vi "Weather Parse Test.vi"() -> ()   [LabVIEW 2020, in "CDM-Config.lvlib"] (continued)
                  \"SUY\"\n                    ]\n                }\n            }\n        },\n        {\n            \"id\": \"https://api.weather.gov/alerts/urn:oid:2.49.0.1.840.0.13e054451602e8337e1efcccba613b86623b52ca.001.1\",\n            \"type\": \"Feature\",\n            \"geometry\": null,\n            \"properties\": {\n                \"@id\": \"https://api.weather.gov/alerts/urn:oid:2.49.0.1.840.0.13e054451602e8337e1efcccba613b86623b52ca.001.1\",\n                \"@type\": \"wx:Alert\",\n                \"id\": \"urn:oid:2.49.0.1.840.0.13e054451602e8337e1efcccba613b86623b52ca.001.1\",\n                \"areaDesc\": \"Cimarron; Texas; Dallam; Sherman; Hansford; Hartley; Moore; Hutchinson; Oldham; Potter; Carson; Deaf Smith; Randall; Armstrong; Palo Duro Canyon\",\n                \"geocode\": {\n                    \"SAME\": [\n                        \"040025\",\n                        \"040139\",\n                        \"048111\",\n                        \"048421\",\n                        \"048195\",\n                        \"048205\",\n                        \"048341\",\n                        \"048233\",\n                        \"048359\",\n                        \"048375\",\n                        \"048065\",\n                        \"048117\",\n                        \"048381\",\n                        \"048011\"\n                    ],\n                    \"UGC\": [\n                        \"OKZ001\",\n                        \"OKZ002\",\n                        \"TXZ001\",\n                        \"TXZ002\",\n                        \"TXZ003\",\n                        \"TXZ006\",\n                        \"TXZ007\",\n                        \"TXZ008\",\n                        \"TXZ011\",\n                        \"TXZ012\",\n                        \"TXZ013\",\n                        \"TXZ016\",\n                        \"TXZ017\",\n                        \"TXZ018\",\n                        \"TXZ317\"\n                    ]\n                },\n                \"affectedZones\": [\n                    \"https://api.weather.gov/zones/forecast/OKZ001\",\n                    \"https://api.weather.gov/zones/forecast/OKZ002\",\n                    \"https://api.weather.gov/zones/forecast/TXZ001\",\n                    \"https://api.weather.gov/zones/forecast/TXZ002\",\n                    \"https://api.weather.gov/zones/forecast/TXZ003\",\n                    \"https://api.weather.gov/zones/forecast/TXZ006\",\n                    \"https://api.weather.gov/zones/forecast/TXZ007\",\n                    \"https://api.weather.gov/zones/forecast/TXZ008\",\n                    \"https://api.weather.gov/zones/forecast/TXZ011\",\n                    \"https://api.weather.gov/zones/forecast/TXZ012\",\n                    \"https://api.weather.gov/zones/forecast/TXZ013\",\n                    \"https://api.weather.gov/zones/forecast/TXZ016\",\n                    \"https://api.weather.gov/zones/forecast/TXZ017\",\n                    \"https://api.weather.gov/zones/forecast/TXZ018\",\n                    \"https://api.weather.gov/zones/forecast/TXZ317\"\n                ],\n                \"references\": [],\n                \"sent\": \"2025-12-02T22:29:00-06:00\",\n                \"effective\": \"2025-12-02T22:29:00-06:00\",\n                \"onset\": \"2025-12-02T22:29:00-06:00\",\n                \"expires\": \"2025-12-03T12:00:00-06:00\",\n                \"ends\": null,\n                \"status\": \"Actual\",\n                \"messageType\": \"Alert\",\n                \"category\": \"Met\",\n                \"severity\": \"Moderate\",\n                \"certainty\": \"Observed\",\n                \"urgency\": \"Expected\",\n                \"event\": \"Special Weather Statement\",\n                \"sender\": \"w-nws.webmaster@noaa.gov\",\n                \"senderName\": \"NWS Amarillo TX\",\n                \"headline\": \"Special Weather Statement issued December 2 at 10:29PM CST by NWS Amarillo TX\",\n                \"description\": \"Winter weather is on the way to the Panhandles Wednesday afternoon\\ninto Thursday. A weather system is expected to move over the Four\\nCorners Wednesday and then track east across New Mexico on\\nWednesday night. Out ahead of this system a strong cold front,\\nassociated with a much larger cold air mass over Canada will bring\\ncold enough temperatures to the Panhandles to allow the\\nprecipitation to be in the form of snow.\\n\\nIt's anticipated that this system will produce some snow bands,\\npossibly a narrow area of snow. These band locations could range\\nfrom the Oklahoma Panhandle down to the southern Texas Panhandle.\\nRight now there's high uncertainty on the location of the snow\\nbands, so much that winter highlights are currently on hold. As\\nthe system approaches and we narrow down the areas that have the\\ngreatest chances of impactful accumulating snow, then we'll add\\nwinter highlights as needed.\\n\\nRight now areas covered in this statement have about a 30 to 60\\npercent chance of receiving at least an inch of snow between\\nWednesday afternoon, and Thursday evening. But if these turn out\\nto be narrow snow bands, then there could be several areas that\\nreceive little to no snow, while more isolated areas pick up 1 to\\n2 inches of snow. And those same areas would have about a 10\\npercent chance of greater than 2 inches of snow.\\n\\nAs it stands right now the best chance for snow to occur in\\nOklahoma to northwest Texas would be mid day Wednesday through\\nmidnight Wednesday night. West of Amarillo to Guymon has the best\\nchance for snow from 9PM Wednesday through about 6 AM Thursday\\nmorning. And east of that same line would be from 3AM to 3PM\\nThursday.\",\n                \"instruction\": null,\n                \"response\": \"Execute\",\n                \"parameters\": {\n                    \"AWIPSidentifier\": [\n                        \"SPSAMA\"\n                    ],\n                    \"WMOidentifier\": [\n                        \"WWUS84 KAMA 030429\"\n                    ],\n                    \"BLOCKCHANNEL\": [\n                        \"EAS\",\n                        \"NWEM\",\n                        \"CMAS\"\n                    ],\n                    \"EAS-ORG\": [\n                        \"WXR\"\n                    ]\n                },\n                \"scope\": \"Public\",\n                \"code\": \"IPAWSv1.0\",\n                \"language\": \"en-US\",\n                \"web\": \"http://www.weather.gov\",\n                \"eventCode\": {\n                    \"SAME\": [\n                        \"SPS\"\n                    ],\n                    \"NationalWeatherService\": [\n                        \"SPS\"\n                    ]\n                }\n            }\n        },\n        {\n            \"id\": \"https://api.weather.gov/alerts/urn:oid:2.49.0.1.840.0.4a77df2fdf2b5a368cb145dcee20e0db7f971925.002.1\",\n            \"type\": \"Feature\",\n            \"geometry\": null,\n            \"properties\": {\n                \"@id\": \"https://api.weather.gov/alerts/urn:oid:2.49.0.1.840.0.4a77df2fdf2b5a368cb145dcee20e0db7f971925.002.1\",\n                \"@type\": \"wx:Alert\",\n                \"id\": \"urn:oid:2.49.0.1.840.0.4a77df2fdf2b5a368cb145dcee20e0db7f971925.002.1\",\n                \"areaDesc\": \"Majuro\",\n                \"geocode\": {\n                    \"SAME\": [\n                        \"068190\"\n                    ],\n                    \"UGC\": [\n                        \"MHZ002\"\n                    ]\n                },\n                \"affectedZones\": [\n                    \"https://api.weather.gov/zones/forecast/MHZ002\"\n                ],\n                \"references\": [\n                    {\n                        \"@id\": \"https://api.weather.gov/alerts/urn:oid:2.49.0.1.840.0.fd750872e36744c34b2c9a183ece0ba44d257df6.002.1\",\n                        \"identifier\": \"urn:oid:2.49.0.1.840.0.fd750872e36744c34b2c9a183ece0ba44d257df6.002.1\",\n                        \"sender\": \"w-nws.webmaster@noaa.gov\",\n                        \"sent\": \"2025-12-03T02:41:00+10:00\"\n                    }\n                ],\n                \"sent\": \"2025-12-03T14:00:00+10:00\",\n                \"effective\": \"2025-12-03T14:00:00+10:00\",\n                \"onset\": \"2025-12-03T14:00:00+10:00\",\n                \"expires\": \"2025-12-04T04:00:00+10:00\",\n                \"ends\": \"2025-12-05T16:00:00+10:00\",\n                \"status\": \"Actual\",\n                \"messageType\": \"Update\",\n                \"category\": \"Met\",\n                \"severity\": \"Minor\",\n                \"certainty\": \"Likely\",\n                \"urgency\": \"Expected\",\n                \"event\": \"Coastal Flood Statement\",\n                \"sender\": \"w-nws.webmaster@noaa.gov\",\n                \"senderName\": \"NWS Tiyan GU\",\n                \"headline\": \"Coastal Flood Statement issued December 3 at 2:00PM ChST until December 5 at 4:00PM ChST by NWS Tiyan GU\",\n                \"description\": \"* WHAT...Isolated minor coastal flooding.\\n\\n* WHERE...North and east facing shorelines of Majuro.\\n\\n* WHEN...Through Friday afternoon.\\n\\n* IMPACTS...Some water on low lying roads and property.\\n\\n* ADDITIONAL DETAILS...Tide predictions show increasing wave run\\nup across Majuro this week due a combination of the lunar cycle\\nand a north swell from a distant weather system. Isolated minor\\ncoastal flooding is expected through at least Friday afternoon.\",\n                \"instruction\": \"Watch for debris along low-lying shorelines facing north and\\neast. Residents living along these low-lying shorelines need to\\nmonitor water levels and take actions to protect property from\\ninundation.\",\n                \"response\": \"Monitor\",\n                \"parameters\": {\n                    \"AWIPSidentifier\": [\n                        \"CFWPQ1\"\n                    ],\n                    \"WMOidentifier\": [\n                        \"WHPQ41 PGUM 030400\"\n                    ],\n                    \"NWSheadline\": [\n                        \"COASTAL FLOOD STATEMENT REMAINS IN EFFECT THROUGH FRIDAY AFTERNOON\"\n                    ],\n                    \"BLOCKCHANNEL\": [\n                        \"EAS\",\n                        \"NWEM\",\n                        \"CMAS\"\n                    ],\n                    \"VTEC\": [\n                        \"/O.CON.PGUM.CF.S.0005.000000T0000Z-251205T0600Z/\"\n                    ],\n                    \"eventEndingTime\": [\n                        \"2025-12-05T16:00:00+10:00\"\n                    ],\n                    \"expiredReferences\": [\n                        \"w-nws.webmaster@noaa.gov,urn:oid:2.49.0.1.840.0.2957d64b6528fdd549b26b0c52e7b17bd496878e.002.1,2025-12-02T14:18:00+10:00 w-nws.webmaster@noaa.gov,urn:oid:2.49.0.1.840.0.d051583a0fc14d57e91ab759b3686451f43fae66.002.1,2025-12-02T03:10:00+10:00 w-nws.webmaster@noaa.gov,urn:oid:2.49.0.1.840.0.3733fd1269a79576a68bee5bf75b40d4db85707a.002.1,2025-12-01T15:08:00+10:00\"\n                    ]\n                },\n                \"scope\": \"Public\",\n                \"code\": \"IPAWSv1.0\",\n                \"language\": \"en-US\",\n                \"web\": \"http://www.weather.gov\",\n                \"eventCode\": {\n                    \"SAME\": [\n                        \"NWS\"\n                    ],\n                    \"NationalWeatherService\": [\n                        \"CFS\"\n                    ]\n                }\n            }\n        },\n        {\n            \"id\": \"https://api.weather.gov/alerts/urn:oid:2.49.0.1.840.0.4a77df2fdf2b5a368cb145dcee20e0db7f971925.001.1\",\n            \"type\": \"Feature\",\n            \"geometry\": null,\n            \"properties\": {\n                \"@id\": \"https://api.weather.gov/alerts/urn:oid:2.49.0.1.840.0.4a77df2fdf2b5a368cb145dcee20e0db7f971925.001.1\",\n                \"@type\": \"wx:Alert\",\n                \"id\": \"urn:oid:2.49.0.1.840.0.4a77df2fdf2b5a368cb145dcee20e0db7f971925.001.1\",\n                \"areaDesc\": \"Kosrae; Pohnpei\",\n                \"geocode\": {\n                    \"SAME\": [\n                        \"064005\",\n                        \"064040\"\n                    ],\n                    \"UGC\": [\n                        \"FMZ001\",\n                        \"FMZ013\"\n                    ]\n                },\n                \"affectedZones\": [\n                    \"https://api.weather.gov/zones/forecast/FMZ001\",\n                    \"https://api.weather.gov/zones/forecast/FMZ013\"\n                ],\n                \"references\": [\n                    {\n                        \"@id\": \"https://api.weather.gov/alerts/urn:oid:2.49.0.1.840.0.fd750872e36744c34b2c9a183ece0ba44d257df6.001.1\",\n                        \"identifier\": \"urn:oid:2.49.0.1.840.0.fd750872e36744c34b2c9a183ece0ba44d257df6.001.1\",\n                        \"sender\": \"w-nws.webmaster@noaa.gov\",\n                        \"sent\": \"2025-12-03T02:41:00+10:00\"\n                    }\n                ],\n                \"sent\": \"2025-12-03T14:00:00+10:00\",\n                \"effective\": \"2025-12-03T14:00:00+10:00\",\n                \"onset\": \"2025-12-03T14:00:00+10:00\",\n                \"expires\": \"2025-12-04T04:00:00+10:00\",\n                \"ends\": \"2025-12-05T16:00:00+10:00\",\n                \"status\": \"Actual\",\n                \"messageType\": \"Update\",\n                \"category\": \"Met\",\n                \"severity\": \"Minor\",\n                \"certainty\": \"Likely\",\n                \"urgency\": \"Expected\",\n                \"event\": \"High Surf Advisory\",\n                \"sender\": \"w-nws.webmaster@noaa.gov\",\n                \"senderName\": \"NWS Tiyan GU\",\n                \"headline\": \"High Surf Advisory issued December 3 at 2:00PM ChST until December 5 at 4:00PM ChST by NWS Tiyan GU\",\n                \"description\": \"* WHAT...Large breaking waves of 7 to 10 feet.\\n\\n* WHERE...North and east facing reefs of Kosrae. North facing\\nreefs of Pohnpei.\\n\\n* WHEN...Until 4 PM ChST Friday.\\n\\n* IMPACTS...Dangerous swimming and surfing conditions and\\nlocalized beach erosion.\\n\\n* ADDITIONAL DETAILS...A long period northerly swell emanating\\nfrom a distant weather system combined with a large northeast\\ntrade swell continue to produce hazardous surf conditions for\\nPohnpei and Kosrae. Surf conditions look to remain hazardous\\nthrough at least Friday afternoon.\",\n                \"instruction\": \"Inexperienced swimmers should remain out of the water due to\\ndangerous surf conditions.\",\n                \"response\": \"Avoid\",\n                \"parameters\": {\n                    \"AWIPSidentifier\": [\n                        \"CFWPQ1\"\n                    ],\n                    \"WMOidentifier\": [\n                        \"WHPQ41 PGUM 030400\"\n                    ],\n                    \"NWSheadline\": [\n                        \"HIGH SURF ADVISORY NOW IN EFFECT UNTIL 4 PM CHST FRIDAY\"\n                    ],\n                    \"BLOCKCHANNEL\": [\n                        \"EAS\",\n                        \"NWEM\",\n                        \"CMAS\"\n                    ],\n                    \"VTEC\": [\n                        \"/O.EXT.PGUM.SU.Y.0038.000000T0000Z-251205T0600Z/\"\n                    ],\n                    \"eventEndingTime\": [\n                        \"2025-12-05T16:00:00+10:00\"\n                    ],\n                    \"expiredReferences\": [\n                        \"w-nws.webmaster@noaa.gov,urn:oid:2.49.0.1.840.0.2957d64b6528fdd549b26b0c52e7b17bd496878e.001.1,2025-12-02T14:18:00+10:00 w-nws.webmaster@noaa.gov,urn:oid:2.49.0.1.840.0.d051583a0fc14d57e91ab759b3686451f43fae66.001.1,2025-12-02T03:10:00+10:00 w-nws.webmaster@noaa.gov,urn:oid:2.49.0.1.840.0.3733fd1269a79576a68bee5bf75b40d4db85707a.001.1,2025-12-01T15:08:00+10:00\"\n                    ]\n                },\n                \"scope\": \"Public\",\n                \"code\": \"IPAWSv1.0\",\n                \"language\": \"en-US\",\n                \"web\": \"http://www.weather.gov\",\n                \"eventCode\": {\n                    \"SAME\": [\n                        \"NWS\"\n                    ],\n                    \"NationalWeatherService\": [\n                        \"SUY\"\n                    ]\n                }\n            }\n        },\n        {\n            \"id\": \"https://api.weather.gov/alerts/urn:oid:2.49.0.1.840.0.93baf164a8b81bd591d12264ddf37071887c834c.001.1\",\n            \"type\": \"Feature\",\n            \"geometry\": null,\n            \"properties\": {\n                \"@id\": \"https://api.weather.gov/alerts/urn:oid:2.49.0.1.840.0.93baf164a8b81bd591d12264ddf37071887c834c.001.1\",\n                \"@type\": \"wx:Alert\",\n                \"id\": \"urn:oid:2.49.0.1.840.0.93baf164a8b81bd591d12264ddf37071887c834c.001.1\",\n                \"areaDesc\": \"Kuskokwim Valley West; Kuskokwim Valley East; Kuskokwim Delta Coast and Nunivak Island; Interior Kuskokwim Delta\",\n                \"geocode\": {\n                    \"SAME\": [\n                        \"002050\"\n                    ],\n                    \"UGC\": [\n                        \"AKZ752\",\n                        \"AKZ753\",\n                        \"AKZ755\",\n                        \"AKZ756\"\n                    ]\n                },\n                \"affectedZones\": [\n                    \"https://api.weather.gov/zones/forecast/AKZ752\",\n                    \"https://api.weather.gov/zones/forecast/AKZ753\",\n                    \"https://api.weather.gov/zones/forecast/AKZ755\",\n                    \"https://api.weather.gov/zones/forecast/AKZ756\"\n                ],\n                \"references\": [],\n                \"sent\": \"2025-12-02T18:07:00-09:00\",\n                \"effective\": \"2025-12-02T18:07:00-09:00\",\n                \"onset\": \"2025-12-02T18:07:00-09:00\",\n                \"expires\": \"2025-12-03T09:00:00-09:00\",\n                \"ends\": \"2025-12-03T09:00:00-09:00\",\n                \"status\": \"Actual\",\n                \"messageType\": \"Alert\",\n                \"category\": \"Met\",\n                \"severity\": \"Extreme\",\n                \"certainty\": \"Likely\",\n                \"urgency\": \"Expected\",\n                \"event\": \"Ice Storm Warning\",\n                \"sender\": \"w-nws.webmaster@noaa.gov\",\n                \"senderName\": \"NWS Anchorage AK\",\n                \"headline\": \"Ice Storm Warning issued December 2 at 6:07PM AKST until December 3 at 9:00AM AKST by NWS Anchorage AK\",\n                \"description\": \"* WHAT...Significant icing expected. Ice accumulations around three\\nquarters of an inch.\\n\\nBlizzard conditions with wind gusts 45 to 55 mph reducing\\nvisibilities to 1/4 mile or less for coastal communities. Total snow\\naccumulations 6 to 12 inches.\\n\\n* WHERE...Kuskokwim Delta, Kuskokwim Valley, including Bethel,\\nAniak, and Crooked Creek for the Ice Storm.\\n\\nCoastal Kuskokwim Delta, including Nunivak and Nelson Islands for\\nBlizzard conditions.\\n\\n* WHEN...Until 9 AM AKST Wednesday.\\n\\n* IMPACTS...Travel could be very difficult. Surfaces will likely\\nbecome slick and hazardous. Significant ice accumulation may cause\\npower outages.\\n\\n* ADDITIONAL DETAILS...Precipitation will remain all snow north and\\nwest of Bethel. North and west of this line is where the Blizzard\\nconditions are ongoing. South and east of this line is where the\\nfreezing rain and Ice Storm conditions are observed.\",\n                \"instruction\": \"An Ice Storm Warning means significant amounts of ice accumulation\\nwill make travel extremely hazardous. Travel is strongly\\ndiscouraged. If you must travel, keep an extra flashlight, food and\\nwater in your vehicle in case of an emergency. Snapped power lines\\nare also possible.\\n\\nPrepare for possible power outages.\",\n                \"response\": \"Avoid\",\n                \"parameters\": {\n                    \"AWIPSidentifier\": [\n                        \"WSWALU\"\n                    ],\n                    \"WMOidentifier\": [\n                        \"WWAK42 PAFC 030307\"\n                    ],\n                    \"NWSheadline\": [\n                        \"ICE STORM WARNING REMAINS IN EFFECT UNTIL 9 AM AKST WEDNESDAY\"\n                    ],\n                    \"BLOCKCHANNEL\": [\n                        \"EAS\",\n                        \"NWEM\",\n                        \"CMAS\"\n                    ],\n                    \"EAS-ORG\": [\n                        \"WXR\"\n                    ],\n                    \"VTEC\": [\n                        \"/O.CON.PAFC.IS.W.0001.000000T0000Z-251203T1800Z/\"\n                    ],\n                    \"eventEndingTime\": [\n                        \"2025-12-03T09:00:00-09:00\"\n                    ],\n                    \"expiredReferences\": [\n                        \"w-nws.webmaster@noaa.gov,urn:oid:2.49.0.1.840.0.157c6f2e53da98a274a7f19e61fa4d73bdd57178.001.1,2025-12-02T00:42:00-09:00 w-nws.webmaster@noaa.gov,urn:oid:2.49.0.1.840.0.9ea12a385b049ff9ed2921f4adaaa88d8666a4fc.001.1,2025-12-01T15:28:00-09:00 w-nws.webmaster@noaa.gov,urn:oid:2.49.0.1.840.0.06a0cb035223f236a02d184a1ba736560d41ecbc.001.1,2025-12-01T04:08:00-09:00 w-nws.webmaster@noaa.gov,urn:oid:2.49.0.1.840.0.f69cd697e861d099e81d8f76b79e96457dfc9a38.001.1,2025-11-30T21:45:00-09:00 w-nws.webmaster@noaa.gov,urn:oid:2.49.0.1.840.0.ccdfa33bcad75d3bc47e8857a243a2cb5db88702.001.2,2025-11-30T09:50:00-09:00\"\n                    ]\n                },\n                \"scope\": \"Public\",\n                \"code\": \"IPAWSv1.0\",\n                \"language\": \"en-US\",\n                \"web\": \"http://www.weather.gov\",\n                \"eventCode\": {\n                    \"SAME\": [\n                        \"WSW\"\n                    ],\n                    \"NationalWeatherService\": [\n                        \"ISW\"\n                    ]\n                }\n            }\n        },\n        {\n            \"id\": \"https://api.weather.gov/alerts/urn:oid:2.49.0.1.840.0.72e634b4e6e77a16c94a0f4f045ba7b0b7412415.001.1\",\n            \"type\": \"Feature\",\n            \"geometry\": null,\n            \"properties\": {\n                \"@id\": \"https://api.weather.gov/alerts/urn:oid:2.49.0.1.840.0.72e634b4e6e77a16c94a0f4f045ba7b0b7412415.001.1\",\n                \"@type\": \"wx:Alert\",\n                \"id\": \"urn:oid:2.49.0.1.840.0.72e634b4e6e77a16c94a0f4f045ba7b0b7412415.001.1\",\n                \"areaDesc\": \"Yukon Delta Coast; Lower Yukon River; Lower Yukon and Innoko Valleys; North Slopes of the Western Alaska Range; Upper Kuskokwim Valley\",\n                \"geocode\": {\n                    \"SAME\": [\n                        \"002158\",\n                        \"002290\"\n                    ],\n                    \"UGC\": [\n                        \"AKZ825\",\n                        \"AKZ826\",\n                        \"AKZ830\",\n                        \"AKZ851\",\n                        \"AKZ852\"\n                    ]\n                },\n                \"affectedZones\": [\n                    \"https://api.weather.gov/zones/forecast/AKZ825\",\n                    \"https://api.weather.gov/zones/forecast/AKZ826\",\n                    \"https://api.weather.gov/zones/forecast/AKZ830\",\n                    \"https://api.weather.gov/zones/forecast/AKZ851\",\n                    \"https://api.weather.gov/zones/forecast/AKZ852\"\n                ],\n                \"references\": [\n                    {\n                        \"@id\": \"https://api.weather.gov/alerts/urn:oid:2.49.0.1.840.0.34d9addf2f9305801f81e1a30a2fd898a36c56d1.001.1\",\n                        \"identifier\": \"urn:oid:2.49.0.1.840.0.34d9addf2f9305801f81e1a30a2fd898a36c56d1.001.1\",\n                        \"sender\": \"w-nws.webmaster@noaa.gov\",\n                        \"sent\": \"2025-12-02T14:06:00-09:00\"\n                    },\n                    {\n                        \"@id\": \"https://api.weather.gov/alerts/urn:oid:2.49.0.1.840.0.0c7829ccd4c9dcb93f8b1cc70bbc58a8100d270e.002.1\",\n                        \"identifier\": \"urn:oid:2.49.0.1.840.0.0c7829ccd4c9dcb93f8b1cc70bbc58a8100d270e.002.1\",\n                        \"sender\": \"w-nws.webmaster@noaa.gov\",\n                        \"sent\": \"2025-12-02T17:58:00-09:00\"\n                    }\n                ],\n                \"sent\": \"2025-12-02T17:59:00-09:00\",\n                \"effective\": \"2025-12-02T17:59:00-09:00\",\n                \"onset\": \"2025-12-02T17:59:00-09:00\",\n                \"expires\": \"2025-12-03T15:00:00-09:00\",\n                \"ends\": \"2025-12-03T15:00:00-09:00\",\n                \"status\": \"Actual\",\n                \"messageType\": \"Update\",\n                \"category\": \"Met\",\n                \"severity\": \"Severe\",\n                \"certainty\": \"Likely\",\n                \"urgency\": \"Expected\",\n                \"event\": \"Winter Storm Warning\",\n                \"sender\": \"w-nws.webmaster@noaa.gov\",\n                \"senderName\": \"NWS Fairbanks AK\",\n                \"headline\": \"Winter Storm Warning issued December 2 at 5:59PM AKST until December 3 at 3:00PM AKST by NWS Fairbanks AK\",\n                \"description\": \"* WHAT...Heavy mixed precipitation. Additional snow accumulations up\\nto 4 inches and ice accumulations around a light glaze. Winds\\ngusting as high as 40 mph.\\n\\n* WHERE...Lower Yukon River, Lower Yukon and Innoko Valleys, North\\nSlopes of the Western Alaska Range, Upper Kuskokwim Valley, and\\nYukon Delta Coast.\\n\\n* WHEN...Until 3 PM AKST Wednesday.\\n\\n* IMPACTS...Surfaces will likely become slick and hazardous.\\nSignificant ice accumulation may cause power outages. Plan on very\\ndifficult traveling conditions.\\n\\nAdditional Details...\\nPrecipitation will be mainly snow, with a chance of freezing rain\\nlingering from McGrath south to the Alaska Range. Blizzard\\nconditions are expected at times for Hooper Bay and Chevak.\\nPrecipitation will taper off on Wednesday morning. Skies clear and\\ntemperatures cool rapidly Wednesday night.\",\n                \"instruction\": \"If you must travel, keep an extra flashlight, food, and water in\\nyour vehicle in case of an emergency. The latest road conditions for\\nthe state you are calling from can be obtained by calling 5 1 1.\",\n                \"response\": \"Prepare\",\n                \"parameters\": {\n                    \"AWIPSidentifier\": [\n                        \"WSWWCZ\"\n                    ],\n                    \"WMOidentifier\": [\n                        \"WWAK42 PAFG 030259\"\n                    ],\n                    \"NWSheadline\": [\n                        \"WINTER STORM WARNING REMAINS IN EFFECT UNTIL 3 PM AKST WEDNESDAY\"\n                    ],\n                    \"BLOCKCHANNEL\": [\n                        \"EAS\",\n                        \"NWEM\",\n                        \"CMAS\"\n                    ],\n                    \"EAS-ORG\": [\n                        \"WXR\"\n                    ],\n                    \"VTEC\": [\n                        \"/O.CON.PAFG.WS.W.0016.000000T0000Z-251204T0000Z/\"\n                    ],\n                    \"eventEndingTime\": [\n                        \"2025-12-03T15:00:00-09:00\"\n                    ],\n                    \"expiredReferences\": [\n                        \"w-nws.webmaster@noaa.gov,urn:oid:2.49.0.1.840.0.3180dc61ca5a09497ed0209ae9ba5ca85fe9aa38.001.1,2025-12-01T14:18:00-09:00 w-nws.webmaster@noaa.gov,urn:oid:2.49.0.1.840.0.ce7a20a2b61779be608b2c765e4513dcaffa8902.001.1,2025-11-30T21:20:00-09:00 w-nws.webmaster@noaa.gov,urn:oid:2.49.0.1.840.0.9c226504b9ca64cc9a49e8dc3ca9fdc84fc4ba17.001.1,2025-11-30T18:03:00-09:00 w-nws.webmaster@noaa.gov,urn:oid:2.49.0.1.840.0.8f81aa3d43b03a8113b1ac64dd14a9f9aab497bb.001.1,2025-11-30T13:06:00-09:00 w-nws.webmaster@noaa.gov,urn:oid:2.49.0.1.840.0.bf2353bea365d572d4db55ee3da60224ffafc19c.001.1,2025-11-29T15:10:00-09:00 w-nws.webmaster@noaa.gov,urn:oid:2.49.0.1.840.0.7ae26db47c90a11c53b2cafe361544d352e847b0.001.2,2025-11-29T13:57:00-09:00\"\n                    ]\n                },\n                \"scope\": \"Public\",\n                \"code\": \"IPAWSv1.0\",\n                \"language\": \"en-US\",\n                \"web\": \"http://www.weather.gov\",\n                \"eventCode\": {\n                    \"SAME\": [\n                        \"WSW\"\n                    ],\n                    \"NationalWeatherService\": [\n                        \"WSW\"\n                    ]\n                }\n            }\n        },\n        {\n            \"id\": \"https://api.weather.gov/alerts/urn:oid:2.49.0.1.840.0.b000524d144bb9785b0e4255566a1e1b34961a53.002.1\",\n            \"type\": \"Feature\",\n            \"geometry\": null,\n            \"properties\": {\n                \"@id\": \"https://api.weather.gov/alerts/urn:oid:2.49.0.1.840.0.b000524d144bb9785b0e4255566a1e1b34961a53.002.1\",\n                \"@type\": \"wx:Alert\",\n                \"id\": \"urn:oid:2.49.0.1.840.0.b000524d144bb9785b0e4255566a1e1b34961a53.002.1\",\n                \"areaDesc\": \"Delta Junction; Upper Chena River Valley; Tanana Flats; Eielson AFB and Salcha; Goldstream Valley and Nenana Hills; Chatanika River Valley; Two Rivers; Fairbanks Metro Area; Nenana; Central Interior; Northern Denali Borough; Eastern Alaska Range North of Trims Camp\",\n                \"geocode\": {\n                    \"SAME\": [\n                        \"002240\",\n                        \"002090\",\n                        \"002290\",\n                        \"002068\"\n                    ],\n                    \"UGC\": [\n                        \"AKZ837\",\n                        \"AKZ838\",\n                        \"AKZ839\",\n                        \"AKZ840\",\n                        \"AKZ841\",\n                        \"AKZ842\",\n                        \"AKZ843\",\n                        \"AKZ844\",\n                        \"AKZ845\",\n                        \"AKZ846\",\n                        \"AKZ847\",\n                        \"AKZ849\"\n                    ]\n                },\n                \"affectedZones\": [\n                    \"https://api.weather.gov/zones/forecast/AKZ837\",\n                    \"https://api.weather.gov/zones/forecast/AKZ838\",\n                    \"https://api.weather.gov/zones/forecast/AKZ839\",\n                    \"https://api.weather.gov/zones/forecast/AKZ840\",\n                    \"https://api.weather.gov/zones/forecast/AKZ841\",\n                    \"https://api.weather.gov/zones/forecast/AKZ842\",\n                    \"https://api.weather.gov/zones/forecast/AKZ843\",\n                    \"https://api.weather.gov/zones/forecast/AKZ844\",\n                    \"https://api.weather.gov/zones/forecast/AKZ845\",\n                    \"https://api.weather.gov/zones/forecast/AKZ846\",\n                    \"https://api.weather.gov/zones/forecast/AKZ847\",\n                    \"https://api.weather.gov/zones/forecast/AKZ849\"\n                ],\n                \"references\": [\n                    {\n                        \"@id\": \"https://api.weather.gov/alerts/urn:oid:2.49.0.1.840.0.a9adcd2a2f234bb05aa1391eaba57392f5dc053d.002.1\",\n                        \"identifier\": \"urn:oid:2.49.0.1.840.0.a9adcd2a2f234bb05aa1391eaba57392f5dc053d.002.1\",\n                        \"sender\": \"w-nws.webmaster@noaa.gov\",\n                        \"sent\": \"2025-12-02T14:06:00-09:00\"\n                    },\n                    {\n                        \"@id\": \"https://api.weather.gov/alerts/urn:oid:2.49.0.1.840.0.c87006556e01e6d2311ccd4e96a18bcc4f84c2a1.002.1\",\n                        \"identifier\": \"urn:oid:2.49.0.1.840.0.c87006556e01e6d2311ccd4e96a18bcc4f84c2a1.002.1\",\n                        \"sender\": \"w-nws.webmaster@noaa.gov\",\n                        \"sent\": \"2025-12-02T17:58:00-09:00\"\n                    }\n                ],\n                \"sent\": \"2025-12-02T17:59:00-09:00\",\n                \"effective\": \"2025-12-02T17:59:00-09:00\",\n                \"onset\": \"2025-12-02T17:59:00-09:00\",\n                \"expires\": \"2025-12-03T15:00:00-09:00\",\n                \"ends\": \"2025-12-03T15:00:00-09:00\",\n                \"status\": \"Actual\",\n                \"messageType\": \"Update\",\n                \"category\": \"Met\",\n                \"severity\": \"Moderate\",\n                \"certainty\": \"Likely\",\n                \"urgency\": \"Expected\",\n                \"event\": \"Winter Weather Advisory\",\n                \"sender\": \"w-nws.webmaster@noaa.gov\",\n                \"senderName\": \"NWS Fairbanks AK\",\n                \"headline\": \"Winter Weather Advisory issued December 2 at 5:59PM AKST until December 3 at 3:00PM AKST by NWS Fairbanks AK\",\n                \"description\": \"* WHAT...Mixed precipitation. Additional snow accumulations up to 4\\ninches and ice accumulations around a light glaze.\\n\\n* WHERE...Central Interior and Northern Alaska Range.\\n\\n* WHEN...Until 3 PM AKST Wednesday.\\n\\n* IMPACTS...Plan on slippery road conditions. Travel may be\\ndifficult.\\n\\nAdditional Details...\\n- Highest snow amounts will be near Tanana, north of Fairbanks\\ntowards Chatanika and along Chena Hot Springs Road east of Two\\nRivers.\\n- Wind gusts as high as 60 mph in Isabel Pass, north of Trims Camp\\nthrough Tuesday night.\",\n                \"instruction\": \"Slow down and use caution while traveling. The latest road\\nconditions for the state you are calling from can be obtained by\\ncalling 5 1 1.\",\n                \"response\": \"Execute\",\n                \"parameters\": {\n                    \"AWIPSidentifier\": [\n                        \"WSWAFG\"\n                    ],\n                    \"WMOidentifier\": [\n                        \"WWAK43 PAFG 030259\"\n                    ],\n                    \"NWSheadline\": [\n                        \"WINTER WEATHER ADVISORY REMAINS IN EFFECT UNTIL 3 PM AKST WEDNESDAY\"\n                    ],\n                    \"BLOCKCHANNEL\": [\n                        \"EAS\",\n                        \"NWEM\",\n                        \"CMAS\"\n                    ],\n                    \"VTEC\": [\n                        \"/O.CON.PAFG.WW.Y.0083.000000T0000Z-251204T0000Z/\"\n                    ],\n                    \"eventEndingTime\": [\n                        \"2025-12-03T15:00:00-09:00\"\n                    ],\n                    \"expiredReferences\": [\n                        \"w-nws.webmaster@noaa.gov,urn:oid:2.49.0.1.840.0.d284f949d6a931dfb333aeac1d9b0238980b9a42.002.1,2025-12-01T14:18:00-09:00 w-nws.webmaster@noaa.gov,urn:oid:2.49.0.1.840.0.127b22ad6a616670ed5ca00d96a96b0447e1be86.002.1,2025-11-30T21:20:00-09:00 w-nws.webmaster@noaa.gov,urn:oid:2.49.0.1.840.0.8523038346d793d84fde28967b729d0dbcbfd792.002.1,2025-11-30T18:03:00-09:00 w-nws.webmaster@noaa.gov,urn:oid:2.49.0.1.840.0.18b86de8c83305b98ef7d093ad66e21a7c92a76f.003.1,2025-11-30T13:06:00-09:00 w-nws.webmaster@noaa.gov,urn:oid:2.49.0.1.840.0.1b0fda3d8aaf3153dee0424772a3cb33cbe62105.003.1,2025-11-29T15:10:00-09:00\"\n                    ]\n                },\n                \"scope\": \"Public\",\n                \"code\": \"IPAWSv1.0\",\n                \"language\": \"en-US\",\n                \"web\": \"http://www.weather.gov\",\n                \"eventCode\": {\n                    \"SAME\": [\n                        \"NWS\"\n                    ],\n                    \"NationalWeatherService\": [\n                        \"WWY\"\n                    ]\n                }\n            }\n        },\n        {\n            \"id\": \"https://api.weather.gov/alerts/urn:oid:2.49.0.1.840.0.72e634b4e6e77a16c94a0f4f045ba7b0b7412415.003.1\",\n            \"type\": \"Feature\",\n            \"geometry\": null,\n            \"properties\": {\n                \"@id\": \"https://api.weather.gov/alerts/urn:oid:2.49.0.1.840.0.72e634b4e6e77a16c94a0f4f045ba7b0b7412415.003.1\",\n                \"@type\": \"wx:Alert\",\n                \"id\": \"urn:oid:2.49.0.1.840.0.72e634b4e6e77a16c94a0f4f045ba7b0b7412415.003.1\",\n                \"areaDesc\": \"Middle Yukon Valley\",\n                \"geocode\": {\n                    \"SAME\": [\n                        \"002290\"\n                    ],\n                    \"UGC\": [\n                        \"AKZ829\"\n                    ]\n                },\n                \"affectedZones\": [\n                    \"https://api.weather.gov/zones/forecast/AKZ829\"\n                ],\n                \"references\": [\n                    {\n                        \"@id\": \"https://api.weather.gov/alerts/urn:oid:2.49.0.1.840.0.34d9addf2f9305801f81e1a30a2fd898a36c56d1.004.1\",\n                        \"identifier\": \"urn:oid:2.49.0.1.840.0.34d9addf2f9305801f81e1a30a2fd898a36c56d1.004.1\",\n                        \"sender\": \"w-nws.webmaster@noaa.gov\",\n                        \"sent\": \"2025-12-02T14:06:00-09:00\"\n                    },\n                    {\n                        \"@id\": \"https://api.weather.gov/alerts/urn:oid:2.49.0.1.840.0.0c7829ccd4c9dcb93f8b1cc70bbc58a8100d270e.004.1\",\n                        \"identifier\": \"urn:oid:2.49.0.1.840.0.0c7829ccd4c9dcb93f8b1cc70bbc58a8100d270e.004.1\",\n                        \"sender\": \"w-nws.webmaster@noaa.gov\",\n                        \"sent\": \"2025-12-02T17:58:00-09:00\"\n                    }\n                ],\n                \"sent\": \"2025-12-02T17:59:00-09:00\",\n                \"effective\": \"2025-12-02T17:59:00-09:00\",\n                \"onset\": \"2025-12-02T17:59:00-09:00\",\n                \"expires\": \"2025-12-03T15:00:00-09:00\",\n                \"ends\": \"2025-12-03T15:00:00-09:00\",\n                \"status\": \"Actual\",\n                \"messageType\": \"Update\",\n                \"category\": \"Met\",\n                \"severity\": \"Moderate\",\n                \"certainty\": \"Likely\",\n                \"urgency\": \"Expected\",\n                \"event\": \"Winter Weather Advisory\",\n                \"sender\": \"w-nws.webmaster@noaa.gov\",\n                \"senderName\": \"NWS Fairbanks AK\",\n                \"headline\": \"Winter Weather Advisory issued December 2 at 5:59PM AKST until December 3 at 3:00PM AKST by NWS Fairbanks AK\",\n                \"description\": \"* WHAT...Snow. Additional snow accumulations up to 4 inches. Winds\\ngusting as high as 35 mph.\\n\\n* WHERE...Middle Yukon Valley.\\n\\n* WHEN...Until 3 PM AKST Wednesday.\\n\\n* IMPACTS...Travel could be very difficult.\",\n                \"instruction\": \"Slow down and use caution while traveling. The latest road\\nconditions for the state you are calling from can be obtained by\\ncalling 5 1 1.\",\n                \"response\": \"Execute\",\n                \"parameters\": {\n                    \"AWIPSidentifier\": [\n                        \"WSWWCZ\"\n                    ],\n                    \"WMOidentifier\": [\n                        \"WWAK42 PAFG 030259\"\n                    ],\n                    \"NWSheadline\": [\n                        \"WINTER WEATHER ADVISORY REMAINS IN EFFECT UNTIL 3 PM AKST WEDNESDAY\"\n                    ],\n                    \"BLOCKCHANNEL\": [\n                        \"EAS\",\n                        \"NWEM\",\n                        \"CMAS\"\n                    ],\n                    \"VTEC\": [\n                        \"/O.CON.PAFG.WW.Y.0083.000000T0000Z-251204T0000Z/\"\n                    ],\n                    \"eventEndingTime\": [\n                        \"2025-12-03T15:00:00-09:00\"\n                    ],\n                    \"expiredReferences\": [\n                        \"w-nws.webmaster@noaa.gov,urn:oid:2.49.0.1.840.0.3180dc61ca5a09497ed0209ae9ba5ca85fe9aa38.004.1,2025-12-01T14:18:00-09:00 w-nws.webmaster@noaa.gov,urn:oid:2.49.0.1.840.0.ce7a20a2b61779be608b2c765e4513dcaffa8902.004.1,2025-11-30T21:20:00-09:00 w-nws.webmaster@noaa.gov,urn:oid:2.49.0.1.840.0.9c226504b9ca64cc9a49e8dc3ca9fdc84fc4ba17.003.1,2025-11-30T18:03:00-09:00 w-nws.webmaster@noaa.gov,urn:oid:2.49.0.1.840.0.8f81aa3d43b03a8113b1ac64dd14a9f9aab497bb.003.1,2025-11-30T13:06:00-09:00 w-nws.webmaster@noaa.gov,urn:oid:2.49.0.1.840.0.bf2353bea365d572d4db55ee3da60224ffafc19c.003.1,2025-11-29T15:10:00-09:00\"\n                    ]\n                },\n                \"scope\": \"Public\",\n                \"code\": \"IPAWSv1.0\",\n                \"language\": \"en-US\",\n                \"web\": \"http://www.weather.gov\",\n                \"eventCode\": {\n                    \"SAME\": [\n                        \"NWS\"\n                    ],\n                    \"NationalWeatherService\": [\n                        \"WWY\"\n                    ]\n                }\n            }\n        },\n        {\n            \"id\": \"https://api.weather.gov/alerts/urn:oid:2.49.0.1.840.0.72e634b4e6e77a16c94a0f4f045ba7b0b7412415.002.1\",\n            \"type\": \"Feature\",\n            \"geometry\": null,\n            \"properties\": {\n                \"@id\": \"https://api.weather.gov/alerts/urn:oid:2.49.0.1.840.0.72e634b4e6e77a16c94a0f4f045ba7b0b7412415.002.1\",\n                \"@type\": \"wx:Alert\",\n                \"id\": \"urn:oid:2.49.0.1.840.0.72e634b4e6e77a16c94a0f4f045ba7b0b7412415.002.1\",\n                \"areaDesc\": \"Eastern Norton Sound and Nulato Hills\",\n                \"geocode\": {\n                    \"SAME\": [\n                        \"002180\"\n                    ],\n                    \"UGC\": [\n                        \"AKZ824\"\n                    ]\n                },\n                \"affectedZones\": [\n                    \"https://api.weather.gov/zones/forecast/AKZ824\"\n                ],\n                \"references\": [\n                    {\n                        \"@id\": \"https://api.weather.gov/alerts/urn:oid:2.49.0.1.840.0.34d9addf2f9305801f81e1a30a2fd898a36c56d1.003.1\",\n                        \"identifier\": \"urn:oid:2.49.0.1.840.0.34d9addf2f9305801f81e1a30a2fd898a36c56d1.003.1\",\n                        \"sender\": \"w-nws.webmaster@noaa.gov\",\n                        \"sent\": \"2025-12-02T14:06:00-09:00\"\n                    },\n                    {\n                        \"@id\": \"https://api.weather.gov/alerts/urn:oid:2.49.0.1.840.0.0c7829ccd4c9dcb93f8b1cc70bbc58a8100d270e.003.1\",\n                        \"identifier\": \"urn:oid:2.49.0.1.840.0.0c7829ccd4c9dcb93f8b1cc70bbc58a8100d270e.003.1\",\n                        \"sender\": \"w-nws.webmaster@noaa.gov\",\n                        \"sent\": \"2025-12-02T17:58:00-09:00\"\n                    }\n                ],\n                \"sent\": \"2025-12-02T17:59:00-09:00\",\n                \"effective\": \"2025-12-02T17:59:00-09:00\",\n                \"onset\": \"2025-12-02T17:59:00-09:00\",\n                \"expires\": \"2025-12-03T15:00:00-09:00\",\n                \"ends\": \"2025-12-03T15:00:00-09:00\",\n                \"status\": \"Actual\",\n                \"messageType\": \"Update\",\n                \"category\": \"Met\",\n                \"severity\": \"Moderate\",\n                \"certainty\": \"Likely\",\n                \"urgency\": \"Expected\",\n                \"event\": \"Winter Weather Advisory\",\n                \"sender\": \"w-nws.webmaster@noaa.gov\",\n                \"senderName\": \"NWS Fairbanks AK\",\n                \"headline\": \"Winter Weather Advisory issued December 2 at 5:59PM AKST until December 3 at 3:00PM AKST by NWS Fairbanks AK\",\n                \"description\": \"* WHAT...Snow. Additional snow accumulations up to two inches. Winds\\ngusting as high as 40 mph.\\n\\n* WHERE...Eastern Norton Sound and Nulato Hills south of Shaktoolik.\\n\\n* WHEN...Until 3 PM AKST Wednesday.\\n\\n* IMPACTS...Travel could be very difficult. The band of snow will\\nshift north Tuesday afternoon and evening, and Unalakleet will\\nlikely see a brief period of poor conditions between 4pm and\\nmidnight. Shaktoolik will remain windy, but snow is not expected.\",\n                \"instruction\": \"Slow down and use caution while traveling. The latest road\\nconditions for the state you are calling from can be obtained by\\ncalling 5 1 1.\",\n                \"response\": \"Execute\",\n                \"parameters\": {\n                    \"AWIPSidentifier\": [\n                        \"WSWWCZ\"\n                    ],\n                    \"WMOidentifier\": [\n                        \"WWAK42 PAFG 030259\"\n                    ],\n                    \"NWSheadline\": [\n                        \"WINTER WEATHER ADVISORY REMAINS IN EFFECT UNTIL 3 PM AKST WEDNESDAY\"\n                    ],\n                    \"BLOCKCHANNEL\": [\n                        \"EAS\",\n                        \"NWEM\",\n                        \"CMAS\"\n                    ],\n                    \"VTEC\": [\n                        \"/O.CON.PAFG.WW.Y.0083.000000T0000Z-251204T0000Z/\"\n                    ],\n                    \"eventEndingTime\": [\n                        \"2025-12-03T15:00:00-09:00\"\n                    ],\n                    \"expiredReferences\": [\n                        \"w-nws.webmaster@noaa.gov,urn:oid:2.49.0.1.840.0.3180dc61ca5a09497ed0209ae9ba5ca85fe9aa38.003.1,2025-12-01T14:18:00-09:00 w-nws.webmaster@noaa.gov,urn:oid:2.49.0.1.840.0.ce7a20a2b61779be608b2c765e4513dcaffa8902.003.1,2025-11-30T21:20:00-09:00 w-nws.webmaster@noaa.gov,urn:oid:2.49.0.1.840.0.9c226504b9ca64cc9a49e8dc3ca9fdc84fc4ba17.002.1,2025-11-30T18:03:00-09:00 w-nws.webmaster@noaa.gov,urn:oid:2.49.0.1.840.0.8f81aa3d43b03a8113b1ac64dd14a9f9aab497bb.002.1,2025-11-30T13:06:00-09:00 w-nws.webmaster@noaa.gov,urn:oid:2.49.0.1.840.0.bf2353bea365d572d4db55ee3da60224ffafc19c.002.1,2025-11-29T15:10:00-09:00\"\n                    ]\n                },\n                \"scope\": \"Public\",\n                \"code\": \"IPAWSv1.0\",\n                \"language\": \"en-US\",\n                \"web\": \"http://www.weather.gov\",\n                \"eventCode\": {\n                    \"SAME\": [\n                        \"NWS\"\n                    ],\n                    \"NationalWeatherService\": [\n                        \"WWY\"\n                    ]\n                }\n            }\n        },\n        {\n            \"id\": \"https://api.weather.gov/alerts/urn:oid:2.49.0.1.840.0.b000524d144bb9785b0e4255566a1e1b34961a53.001.1\",\n            \"type\": \"Feature\",\n            \"geometry\": null,\n            \"properties\": {\n                \"@id\": \"https://api.weather.gov/alerts/urn:oid:2.49.0.1.840.0.b000524d144bb9785b0e4255566a1e1b34961a53.001.1\",\n                \"@type\": \"wx:Alert\",\n                \"id\": \"urn:oid:2.49.0.1.840.0.b000524d144bb9785b0e4255566a1e1b34961a53.001.1\",\n                \"areaDesc\": \"Dalton Highway Summits; Yukon Flats; White Mountains and High Terrain South of the Yukon River; Fortymile Country\",\n                \"geocode\": {\n                    \"SAME\": [\n                        \"002290\",\n                        \"002240\"\n                    ],\n                    \"UGC\": [\n                        \"AKZ832\",\n                        \"AKZ833\",\n                        \"AKZ834\",\n                        \"AKZ835\"\n                    ]\n                },\n                \"affectedZones\": [\n                    \"https://api.weather.gov/zones/forecast/AKZ832\",\n                    \"https://api.weather.gov/zones/forecast/AKZ833\",\n                    \"https://api.weather.gov/zones/forecast/AKZ834\",\n                    \"https://api.weather.gov/zones/forecast/AKZ835\"\n                ],\n                \"references\": [\n                    {\n                        \"@id\": \"https://api.weather.gov/alerts/urn:oid:2.49.0.1.840.0.a9adcd2a2f234bb05aa1391eaba57392f5dc053d.001.1\",\n                        \"identifier\": \"urn:oid:2.49.0.1.840.0.a9adcd2a2f234bb05aa1391eaba57392f5dc053d.001.1\",\n                        \"sender\": \"w-nws.webmaster@noaa.gov\",\n                        \"sent\": \"2025-12-02T14:06:00-09:00\"\n                    },\n                    {\n                        \"@id\": \"https://api.weather.gov/alerts/urn:oid:2.49.0.1.840.0.c87006556e01e6d2311ccd4e96a18bcc4f84c2a1.001.1\",\n                        \"identifier\": \"urn:oid:2.49.0.1.840.0.c87006556e01e6d2311ccd4e96a18bcc4f84c2a1.001.1\",\n                        \"sender\": \"w-nws.webmaster@noaa.gov\",\n                        \"sent\": \"2025-12-02T17:58:00-09:00\"\n                    }\n                ],\n                \"sent\": \"2025-12-02T17:59:00-09:00\",\n                \"effective\": \"2025-12-02T17:59:00-09:00\",\n                \"onset\": \"2025-12-02T17:59:00-09:00\",\n                \"expires\": \"2025-12-03T15:00:00-09:00\",\n                \"ends\": \"2025-12-03T15:00:00-09:00\",\n                \"status\": \"Actual\",\n                \"messageType\": \"Update\",\n                \"category\": \"Met\",\n                \"severity\": \"Moderate\",\n                \"certainty\": \"Likely\",\n                \"urgency\": \"Expected\",\n                \"event\": \"Winter Weather Advisory\",\n                \"sender\": \"w-nws.webmaster@noaa.gov\",\n                \"senderName\": \"NWS Fairbanks AK\",\n                \"headline\": \"Winter Weather Advisory issued December 2 at 5:59PM AKST until December 3 at 3:00PM AKST by NWS Fairbanks AK\",\n                \"description\": \"* WHAT...Snow. Additional snow accumulations up to 4 inches.\\n\\n* WHERE...Dalton Highway Summits, Yukon Uplands, White Mountains and\\nHigh Terrain South of the Yukon River, and Yukon Flats.\\n\\n* WHEN...Until 3 PM AKST Wednesday.\\n\\n* IMPACTS...Travel could be very difficult. The highest snow amounts\\nwill be in the White Mountains and Steese Highway Summits.\",\n                \"instruction\": \"Slow down and use caution while traveling. The latest road\\nconditions for the state you are calling from can be obtained by\\ncalling 5 1 1.\",\n                \"response\": \"Execute\",\n                \"parameters\": {\n                    \"AWIPSidentifier\": [\n                        \"WSWAFG\"\n                    ],\n                    \"WMOidentifier\": [\n                        \"WWAK43 PAFG 030259\"\n                    ],\n                    \"NWSheadline\": [\n                        \"WINTER WEATHER ADVISORY REMAINS IN EFFECT UNTIL 3 PM AKST WEDNESDAY\"\n                    ],\n                    \"BLOCKCHANNEL\": [\n                        \"EAS\",\n                        \"NWEM\",\n                        \"CMAS\"\n                    ],\n                    \"VTEC\": [\n                        \"/O.CON.PAFG.WW.Y.0083.000000T0000Z-251204T0000Z/\"\n                    ],\n                    \"eventEndingTime\": [\n                        \"2025-12-03T15:00:00-09:00\"\n                    ],\n                    \"expiredReferences\": [\n                        \"w-nws.webmaster@noaa.gov,urn:oid:2.49.0.1.840.0.d284f949d6a931dfb333aeac1d9b0238980b9a42.001.1,2025-12-01T14:18:00-09:00 w-nws.webmaster@noaa.gov,urn:oid:2.49.0.1.840.0.127b22ad6a616670ed5ca00d96a96b0447e1be86.001.1,2025-11-30T21:20:00-09:00 w-nws.webmaster@noaa.gov,urn:oid:2.49.0.1.840.0.8523038346d793d84fde28967b729d0dbcbfd792.001.1,2025-11-30T18:03:00-09:00 w-nws.webmaster@noaa.gov,urn:oid:2.49.0.1.840.0.18b86de8c83305b98ef7d093ad66e21a7c92a76f.002.1,2025-11-30T13:06:00-09:00 w-nws.webmaster@noaa.gov,urn:oid:2.49.0.1.840.0.1b0fda3d8aaf3153dee0424772a3cb33cbe62105.002.1,2025-11-29T15:10:00-09:00\"\n                    ]\n                },\n                \"scope\": \"Public\",\n                \"code\": \"IPAWSv1.0\",\n                \"language\": \"en-US\",\n                \"web\": \"http://www.weather.gov\",\n                \"eventCode\": {\n                    \"SAME\": [\n                        \"NWS\"\n                    ],\n                    \"NationalWeatherService\": [\n                        \"WWY\"\n                    ]\n                }\n            }\n        },\n        {\n            \"id\": \"https://api.weather.gov/alerts/urn:oid:2.49.0.1.840.0.b000524d144bb9785b0e4255566a1e1b34961a53.003.1\",\n            \"type\": \"Feature\",\n            \"geometry\": null,\n            \"properties\": {\n                \"@id\": \"https://api.weather.gov/alerts/urn:oid:2.49.0.1.840.0.b000524d144bb9785b0e4255566a1e1b34961a53.003.1\",\n                \"@type\": \"wx:Alert\",\n                \"id\": \"urn:oid:2.49.0.1.840.0.b000524d144bb9785b0e4255566a1e1b34961a53.003.1\",\n                \"areaDesc\": \"Southern Denali Borough; Eastern Alaska Range South of Trims Camp\",\n                \"geocode\": {\n                    \"SAME\": [\n                        \"002068\",\n                        \"002240\"\n                    ],\n                    \"UGC\": [\n                        \"AKZ848\",\n                        \"AKZ850\"\n                    ]\n                },\n                \"affectedZones\": [\n                    \"https://api.weather.gov/zones/forecast/AKZ848\",\n                    \"https://api.weather.gov/zones/forecast/AKZ850\"\n                ],\n                \"references\": [\n                    {\n                        \"@id\": \"https://api.weather.gov/alerts/urn:oid:2.49.0.1.840.0.a9adcd2a2f234bb05aa1391eaba57392f5dc053d.003.1\",\n                        \"identifier\": \"urn:oid:2.49.0.1.840.0.a9adcd2a2f234bb05aa1391eaba57392f5dc053d.003.1\",\n                        \"sender\": \"w-nws.webmaster@noaa.gov\",\n                        \"sent\": \"2025-12-02T14:06:00-09:00\"\n                    },\n                    {\n                        \"@id\": \"https://api.weather.gov/alerts/urn:oid:2.49.0.1.840.0.c87006556e01e6d2311ccd4e96a18bcc4f84c2a1.003.1\",\n                        \"identifier\": \"urn:oid:2.49.0.1.840.0.c87006556e01e6d2311ccd4e96a18bcc4f84c2a1.003.1\",\n                        \"sender\": \"w-nws.webmaster@noaa.gov\",\n                        \"sent\": \"2025-12-02T17:58:00-09:00\"\n                    }\n                ],\n                \"sent\": \"2025-12-02T17:59:00-09:00\",\n                \"effective\": \"2025-12-02T17:59:00-09:00\",\n                \"onset\": \"2025-12-02T17:59:00-09:00\",\n                \"expires\": \"2025-12-03T15:00:00-09:00\",\n                \"ends\": \"2025-12-03T15:00:00-09:00\",\n                \"status\": \"Actual\",\n                \"messageType\": \"Update\",\n                \"category\": \"Met\",\n                \"severity\": \"Moderate\",\n                \"certainty\": \"Likely\",\n                \"urgency\": \"Expected\",\n                \"event\": \"Winter Weather Advisory\",\n                \"sender\": \"w-nws.webmaster@noaa.gov\",\n                \"senderName\": \"NWS Fairbanks AK\",\n                \"headline\": \"Winter Weather Advisory issued December 2 at 5:59PM AKST until December 3 at 3:00PM AKST by NWS Fairbanks AK\",\n                \"description\": \"* WHAT...Snow. Additional snow accumulations up to 5 inches. Winds\\ngusting as high as 45 mph.\\n\\n* WHERE...Eastern Alaska Range South of Trims Camp and Southern\\nDenali Borough.\\n\\n* WHEN...Until 3 PM AKST Wednesday.\\n\\n* IMPACTS...Travel could be very difficult.\",\n                \"instruction\": \"Slow down and use caution while traveling. The latest road\\nconditions for the state you are calling from can be obtained by\\ncalling 5 1 1.\",\n                \"response\": \"Execute\",\n                \"parameters\": {\n                    \"AWIPSidentifier\": [\n                        \"WSWAFG\"\n                    ],\n                    \"WMOidentifier\": [\n                        \"WWAK43 PAFG 030259\"\n                    ],\n                    \"NWSheadline\": [\n                        \"WINTER WEATHER ADVISORY REMAINS IN EFFECT UNTIL 3 PM AKST WEDNESDAY\"\n                    ],\n                    \"BLOCKCHANNEL\": [\n                        \"EAS\",\n                        \"NWEM\",\n                        \"CMAS\"\n                    ],\n                    \"VTEC\": [\n                        \"/O.CON.PAFG.WW.Y.0083.000000T0000Z-251204T0000Z/\"\n                    ],\n                    \"eventEndingTime\": [\n                        \"2025-12-03T15:00:00-09:00\"\n                    ],\n                    \"expiredReferences\": [\n                        \"w-nws.webmaster@noaa.gov,urn:oid:2.49.0.1.840.0.d284f949d6a931dfb333aeac1d9b0238980b9a42.003.1,2025-12-01T14:18:00-09:00 w-nws.webmaster@noaa.gov,urn:oid:2.49.0.1.840.0.127b22ad6a616670ed5ca00d96a96b0447e1be86.003.1,2025-11-30T21:20:00-09:00 w-nws.webmaster@noaa.gov,urn:oid:2.49.0.1.840.0.8523038346d793d84fde28967b729d0dbcbfd792.003.1,2025-11-30T18:03:00-09:00 w-nws.webmaster@noaa.gov,urn:oid:2.49.0.1.840.0.18b86de8c83305b98ef7d093ad66e21a7c92a76f.001.1,2025-11-30T13:06:00-09:00 w-nws.webmaster@noaa.gov,urn:oid:2.49.0.1.840.0.1b0fda3d8aaf3153dee0424772a3cb33cbe62105.001.1,2025-11-29T15:10:00-09:00\"\n                    ]\n                },\n                \"scope\": \"Public\",\n                \"code\": \"IPAWSv1.0\",\n                \"language\": \"en-US\",\n                \"web\": \"http://www.weather.gov\",\n                \"eventCode\": {\n                    \"SAME\": [\n                        \"NWS\"\n                    ],\n                    \"NationalWeatherService\": [\n                        \"WWY\"\n                    ]\n                }\n            }\n        },\n        {\n            \"id\": \"https://api.weather.gov/alerts/urn:oid:2.49.0.1.840.0.9a5af99817b4d9edcfcd61f0327d754f8de44e19.002.1\",\n            \"type\": \"Feature\",\n            \"geometry\": null,\n            \"properties\": {\n                \"@id\": \"https://api.weather.gov/alerts/urn:oid:2.49.0.1.840.0.9a5af99817b4d9edcfcd61f0327d754f8de44e19.002.1\",\n                \"@type\": \"wx:Alert\",\n                \"id\": \"urn:oid:2.49.0.1.840.0.9a5af99817b4d9edcfcd61f0327d754f8de44e19.002.1\",\n                \"areaDesc\": \"Northern Humboldt Interior; Southern Humboldt Interior\",\n                \"geocode\": {\n                    \"SAME\": [\n                        \"006023\"\n                    ],\n                    \"UGC\": [\n                        \"CAZ105\",\n                        \"CAZ106\"\n                    ]\n                },\n                \"affectedZones\": [\n                    \"https://api.weather.gov/zones/forecast/CAZ105\",\n                    \"https://api.weather.gov/zones/forecast/CAZ106\"\n                ],\n                \"references\": [\n                    {\n                        \"@id\": \"https://api.weather.gov/alerts/urn:oid:2.49.0.1.840.0.572af28717b4d18ac951aaf092ab1eb478907437.001.1\",\n                        \"identifier\": \"urn:oid:2.49.0.1.840.0.572af28717b4d18ac951aaf092ab1eb478907437.001.1\",\n                        \"sender\": \"w-nws.webmaster@noaa.gov\",\n                        \"sent\": \"2025-12-02T10:26:00-08:00\"\n                    }\n                ],\n                \"sent\": \"2025-12-02T18:17:00-08:00\",\n                \"effective\": \"2025-12-02T18:17:00-08:00\",\n            
